vi "Power & Frequency Estimate.vi"(2 "span":i32=7 format="%0.0f", 4 "df":dbl=1.0 format="%0.2f", 5 "window constants":cluster{"eq noise BW":dbl, "coherent gain":dbl}={"eq noise BW"=1.0, "coherent gain"=1.0} {"coherent gain" format="%0.2f"; "eq noise BW" format="%0.2f"}, 6 "peak frequency (max)":dbl=-1.0 format="%0.2f", 7 "Power Spectrum (V^2 rms)":dbl[](array[numeric])) -> (0 "est power peak":dbl format="%0.4f", 1 "est frequency peak":dbl format="%0.4f")   [LabVIEW 2020, in "NI_AALPro.lvlib"]
doc: "Computes the estimated power and frequency around the <B>peak frequency</B> in the power spectrum of a time-domain signal."
uses:
  NI_AALPro.lvlib
panel:
  # "Power and Frequency\nEstimate"
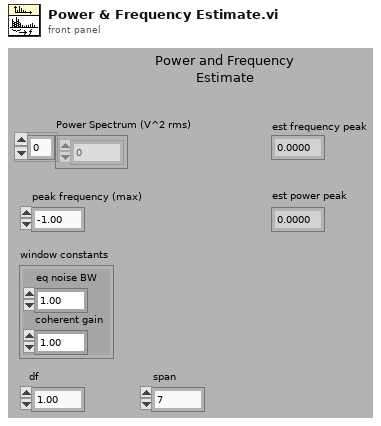
[diagram p1: front panel]
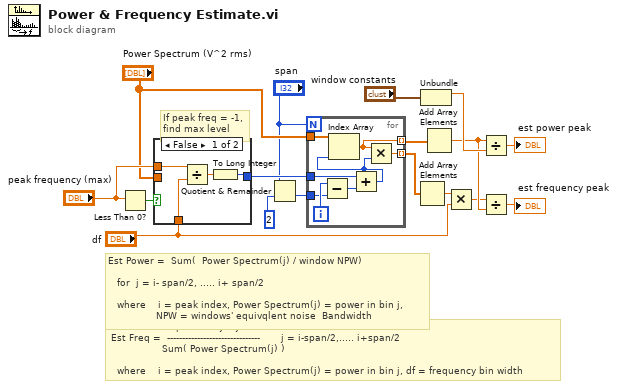
[diagram p0: block diagram]
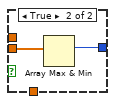
[diagram p2: hidden frame]
diagram:
  # "Sum ( Power Spectrum(j)*(j*df) )                         \n Est Freq =  -------------------------------       j = i-span/2,..... i+span/2\n                  Sum( Power Spectrum(j) )\n\n   where    i = peak index, Power Spectrum(j) = power in bin j, df = frequency bin width"
  # "Est Power =  Sum(  Power Spectrum(j) / window NPW)\n                        \n   for  j = i- span/2, ..... i+ span/2\n\n   where    i = peak index, Power Spectrum(j) = power in bin j, \n                NPW = windows' equivqlent noise  Bandwidth"
  # "If peak freq = -1,\nfind max level"
  n1 = Less Than 0?(x="peak frequency (max)") -> (x < 0?=w15:bool)
  n2 = case shown="False" w15 {
    tunnel: "df" -> [w21 _]
    tunnel: [w18 w22] -> w12
    tunnel: "Power Spectrum (V^2 rms)" -> [_ w23]
    tunnel: "peak frequency (max)" -> [w19 _]
    frame False {
      n3 = Divide(x=w19, y=w21) -> (x/y=w20:dbl)
      n4 = To Long Integer(number=w20) -> (32bit integer=w18:i32)
    }
    frame True {
      n5 = Array Max & Min(array=w23) -> (max index (indices)=w22:i32)  [unwired: 3 out]
    }
  }
  n6 = Quotient & Remainder(x="span", y=2) -> (floor(x/y)=w9:i32)  [unwired: 1 out]
  n7 = for {
    N: "span" -> [_]
    tunnel: [w27] -> w16 mode=indexing
    tunnel: [w24] -> w17 mode=indexing
    tunnel: w12 -> [w28]
    tunnel: w9 -> [w30]
    tunnel: "Power Spectrum (V^2 rms)" -> [w26]
    i -> [w31]
    n8 = Subtract(x=w31, y=w30) -> (x-y=w29:i32)
    n9 = Add(x=w28, y=w29) -> (x+y=w25:i32)
    n10 = Index Array(array=w26, index=w25) -> (element=w24:dbl)
    n11 = Multiply(x=w24, y=w25) -> (x*y=w27:dbl)
  }
  n12 = Add Array Elements(numeric array=w16) -> (sum=w6:dbl)
  n13 = Unbundle("window constants") -> ("eq noise BW"=w4:dbl)  [unwired: 1 out]
  n14 = Add Array Elements(numeric array=w17) -> (sum=w3:dbl)
  n15 = Multiply(x=w6, y="df") -> (x*y=w2:dbl)
  n16 = Divide(x=w3, y=w4) -> (x/y=→"est power peak":dbl)
  n17 = Divide(x=w2, y=w3) -> (x/y=→"est frequency peak":dbl)
